vi "FPGA_start_stop_QPD.vi"(6 "queue FPGA IN":refnum<queue>, 7 "FPGA VI Reference IN":refnum<k20>, 8 "error in":errorcluster, 10 "start ?":bool, 11 "Measuring QPD":bool) -> (0 "error out":errorcluster, 3 "Measuring QPD":bool, 4 "queue FPGA OUT":refnum<queue>, 5 "FPGA VI Reference OUT":refnum<k20>)   [LabVIEW 2015]
uses:
  CONTROLS/Q_FPGA_element.ctl
  <vilib>/FPGAPlugInAG/PCIe-7841R/niLvFpga_Open_PCIe-7841R.vi
  <vilib>/rvi/interface/common/dynamic/niFpgaDynamicAddResources.vi
  <vilib>/Utility/error.llb/Error Cluster From Error Code.vi
  <vilib>/rvi/errors/niLvFpgaAdjustHostInterfaceError.vi
  <vilib>/FPGAPlugInAG/Dynamic/niLvFpga_Run_Dynamic.vi
  <vilib>/FPGAPlugInAG/Dynamic/niLvFpga_Abort_Dynamic.vi
  <vilib>/FPGAPlugInAG/Dynamic/niLvFpga_Close_Dynamic.vi
  <vilib>/rvi/interface/nirviOpenFPGA/nirviOpenFPGA.xnode
  FPGA/FPGA Bitfiles/FPGAv0_FPGATarget_FPGAmeasureQPDsi_91djMVJ3FxY.lvbitx
  <vilib>/rvi/interface/nirviReadWriteControl/nirviReadWriteControl.xnode
  <vilib>/rvi/interface/nirviMethod/nirviMethod.xnode
  <vilib>/rvi/interface/nirviCloseFPGA/nirviCloseFPGA.xnode
  NiFpgaLv.dll
  <vilib>/rvi/interface/Simulation/niFpgaSimulationCallBeginRW.vi
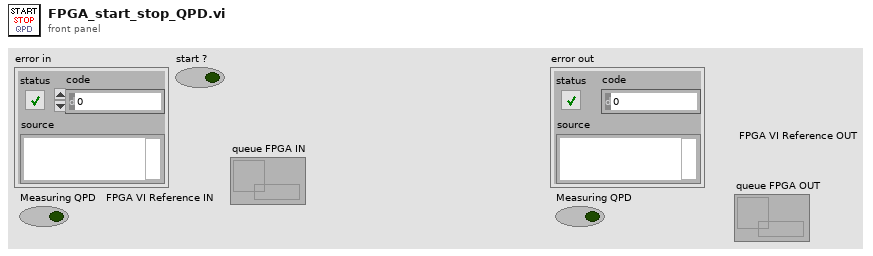
[diagram p1: front panel]
types:
  T1 = typedef "Q_FPGA_element.ctl" = cluster{"variant":variant, "Instruction":enum16{"FPGA_idle", "FPGA_initialize", "FPGA_error", "FPGA_security_stop", "FPGA_laser", "FPGA_start_stop_measure_QPD", "FPGA_measure_QPD", "FPGA_measure_QPD_noise", "FPGA_stop_measure_QPD", "FPGA_init_autofocus", "FPGA_init_single_scan", "FPGA_stop_single_scan", "FPGA_init_merFISH", "FPGA_measure_QPD_merFISH", "FPGA_init_scan_merFISH", "FPGA_scan_merFISH", "FPGA_close_merFISH", "FPGA_stop"}}
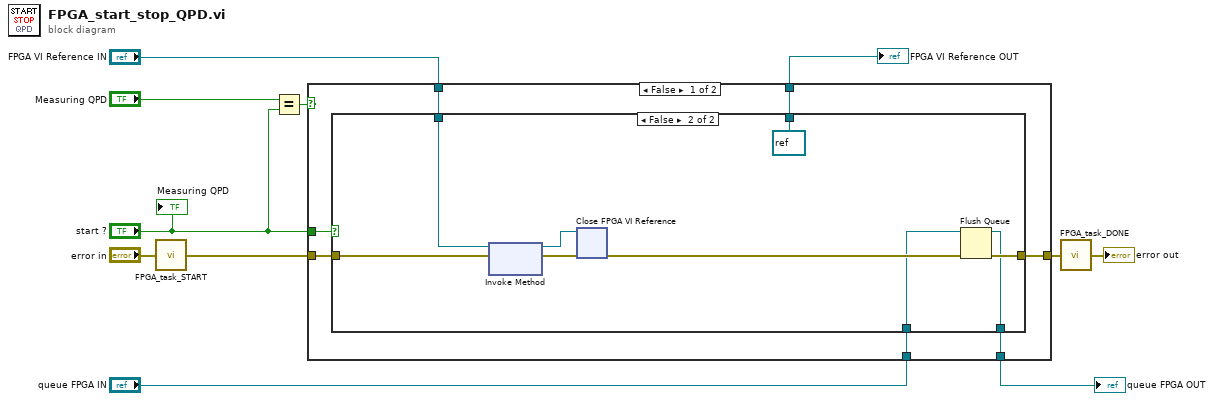
[diagram p0: block diagram]
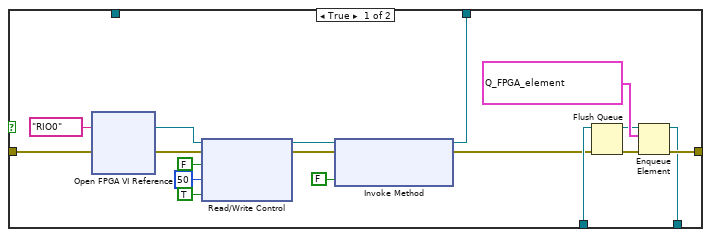
[diagram p2: hidden frame]
diagram:
  n1 = call "FPGA_task_START.vi"("error in"="error in") -> ("error out"=w2:errorcluster)
  n2 = Equal?(x="Measuring QPD", y="start ?") -> (x = y?=w11:bool)
  n3 = case shown="False" w11 {
    tunnel: "queue FPGA IN" -> [w18 w47]
    tunnel: [w17 w47] -> w4
    tunnel: w2 -> [w16 w48]
    tunnel: [w15 w48] -> w10
    tunnel: "start ?" -> [w14 _]
    tunnel: [w13 w46] -> w3
    tunnel: "FPGA VI Reference IN" -> [w12 w46]
    frame False {
      n4 = case shown="False" w14 {
        tunnel: w18 -> [w21 w42]
        tunnel: [w34 w41] -> w15
        tunnel: [w33 w40] -> w17
        tunnel: w16 -> [w31 w37]
        tunnel: [w20 refnum<k20> refnum ("FPGA VI Reference Out")] -> w13
        tunnel: w12 -> [_ w38]
        frame True {
          n5 = xnode ("Open FPGA VI Reference")("error in"=w31, "resource name"=tag "RIO0") -> ("FPGA VI Reference Out"=w29:refnum<k20>, "error out"=w30:errorcluster)
          n6 = xnode "Read/Write Control"("FPGA VI Reference In"=w29, "error in"=w30, "stop"=FALSE, "Count(uSec)"=u32 50, "Reset counter"=TRUE) -> ("FPGA VI Reference Out"=w26:refnum<k20>, "error out"=w28:errorcluster)
          n7 = xnode "Invoke Method"("FPGA VI Reference In"=w26, "error in"=w28, "Wait Until Done (F)"=FALSE) -> ("FPGA VI Reference Out"=w20:refnum<k20>, "error out"=w19:errorcluster)
          n8 = Flush Queue(queue=w21, error in (no error)=w19) -> (queue out=w22:refnum<queue>, error out=w23:errorcluster)  [unwired: 1 out]
          n9 = Enqueue Element(queue=w22, element=T1 {"variant"=variant, "Instruction"=enum."FPGA_measure_QPD"}, error in (no error)=w23) -> (queue out=w33:refnum<queue>, error out=w34:errorcluster)  [unwired: 1 in, 1 out]
        }
        frame False {
          n10 = xnode "Invoke Method"("FPGA VI Reference In"=w38, "error in"=w37) -> ("FPGA VI Reference Out"=w44:refnum<k20>, "error out"=w45:errorcluster)
          n11 = xnode "Close FPGA VI Reference"("FPGA VI Reference In"=w44, "error in"=w45) -> ("error out"=w43:errorcluster)
          n12 = Flush Queue(queue=w42, error in (no error)=w43) -> (queue out=w40:refnum<queue>, error out=w41:errorcluster)  [unwired: 1 out]
        }
      }
    }
    frame True {
    }
  }
  "queue FPGA OUT" <- w4
  "FPGA VI Reference OUT" <- w3
  n13 = call "FPGA_task_DONE.vi"("error in"=w10) -> ("error out"=→"error out":errorcluster)
  "Measuring QPD" <- "start ?"
